vi "Get Prompts.vi"(8 "error in (no error)":errorcluster, 11 "id":i32) -> (0 "error out":errorcluster, 3 "Prompts":T1[](array[typedef]))   [LabVIEW 2025, in "MCP Server.lvlib"]
uses:
  MCP Server.lvlib
  Prompt Data.ctl
  Prompt Argument.ctl
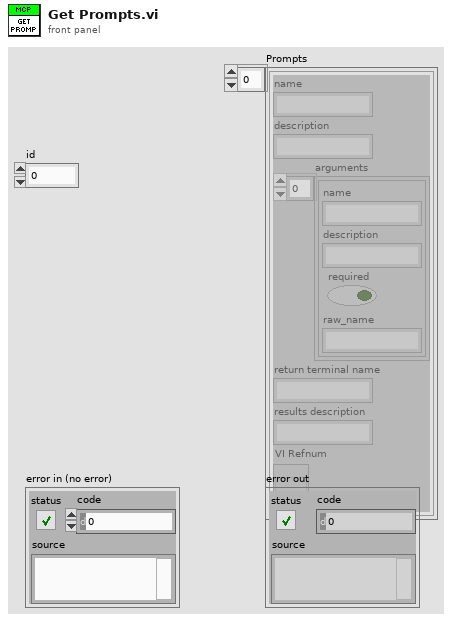
[diagram p1: front panel]
types:
  T1 = typedef "MCP Server.lvlib/Prompt Data.ctl" = cluster{"name":string, "description":string, "arguments":T2[], "return terminal name":string, "results description":string, "VI Refnum":refnum<vi>}
  T2 = typedef "MCP Server.lvlib/Prompt Argument.ctl" = cluster{"name":string, "description":string, "required":bool, "raw_name":string}
  T3 = typedef "MCP Server.lvlib/Server Data.ctl" = cluster{"Name":string, "Description":string, "Tools":T4[], "Parameters":string[][], "Logging Info":T7, "User Events":T8, "Prompts":T1[], "resources":T9[], "HTTP Server":refnum<class "Server.lvclass">}
  T4 = typedef "MCP Server.lvlib/Tool Data.ctl" = cluster{"Name":string, "Description":string, "Ignored":string[], "inputs":T5[], "outputs":T6[], "VI Refnum":refnum<vi>}
  T5 = typedef "MCP Server.lvlib/Input Parameter.ctl" = cluster{"name":string, "type":string, "description":string, "required":bool, "raw name":string}
  T6 = typedef "MCP Server.lvlib/Output Parameter.ctl" = cluster{"name":string, "description":string, "type":string, "raw name":string}
  T7 = typedef "MCP Server.lvlib/Logging.ctl" = cluster{"Log":string[], "Max Length":i32}
  T8 = typedef "MCP Server.lvlib/User Events.ctl" = cluster{"onError":refnum<user-event>, "onRpc":refnum<user-event>}
  T9 = typedef "MCP Server.lvlib/resource data.ctl" = cluster{"uri":string, "name":string, "description":string, "mimeType":string, "file path":path}
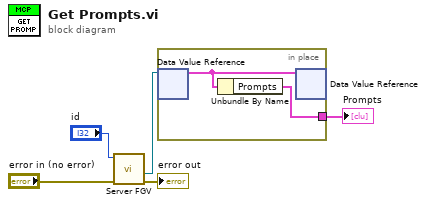
[diagram p0: block diagram]
diagram:
  n1 = call "Server FGV.vi"("error in"="error in (no error)", "id"="id") -> ("error out"=→"error out":errorcluster, "server reference"=w4:refnum<data-value>)  [unwired: 5 in, 3 out]
  n2 = in-place {
    in-place-border: [w7] -> w5
    n3 = in-place-dvr #1(w4) -> (w6:T3)  [unwired: 1 out]
    n4 = Unbundle By Name(w6) -> ("Prompts"=w7:T1[])
    n5 = in-place-dvr #1(w6) -> ()  [unwired: 2 out]
  }
  "Prompts" <- w5
